vi "Image_averaging_FFTW3_test.vi"(0 "buffer in":dbl[][](array[numeric]), 1 "index":dbl[](array[numeric]), 3 "Average":dbl min=0.0 max=1.0 step=0.01, 5 "data":dbl[][](array[numeric]), 7 "# of Cores":i32=3, 9 "input cluster":T1, 11 "error in (no error)":errorcluster, 12 "Soften Image":i32=1, 14 "power":dbl=0.01 min=0.01 max=1.0 step=0.01) -> (4 "buffer out":dbl[][](array[numeric]), 6 "Image":dbl[][](array[numeric]), 10 "complex_depth_profile":dbl[][](array[numeric]), 15 "error out":errorcluster)   [LabVIEW 2017]
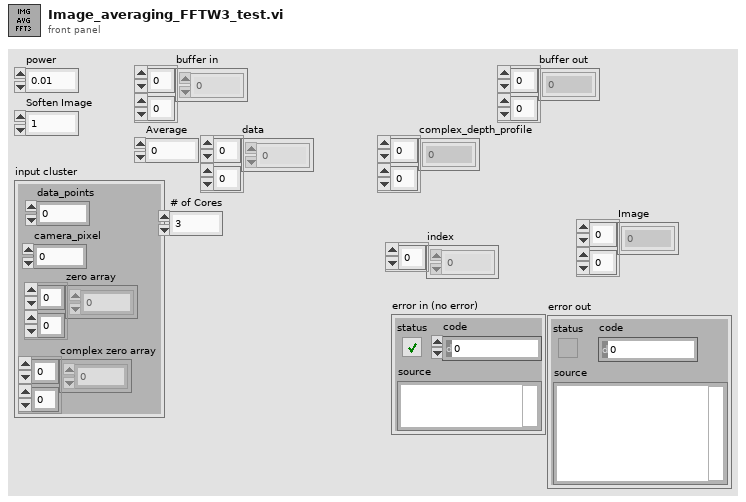
[diagram p1: front panel]
types:
  T1 = cluster{"data_points":i32, "camera_pixel":i32, "zero array":dbl[][], "complex zero array":dbl[][]}
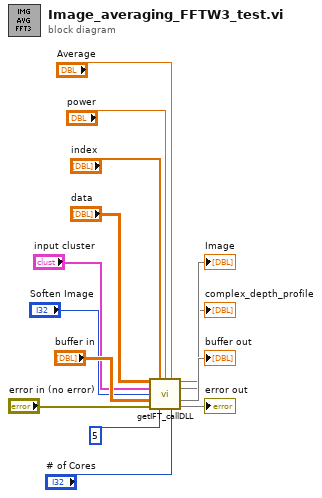
[diagram p0: block diagram]
diagram:
  n1 = call "getIFT_callDLL.vi"(0:"data", 1:"index", 2:"power", 3:"Average", 5:"input cluster", 7:"Soften Image", 9:"buffer in", 11:"error in (no error)", 12:5 ("interp_value"), 14:"# of Cores") -> (4:→"Image", 6:→"complex_depth_profile", 10:→"buffer out", 15:→"error out")  [unwired: 2 in]
